vi "PM100D_Initialize.vi"() -> (0 "error out":errorcluster, 1 "Instrument":string, 2 "VISA out":refnum<visa-resource-name>, 4 "SN":string)   [LabVIEW 2010]
doc: "This VI scans for connected devices, that can be selected in a dialog box. Next steps\n- setting timeout\n- performing identification query\n- configuring the operation register to '512'; flag gets to HI when a new measurement value is ready to fetch\n- clear operation register"
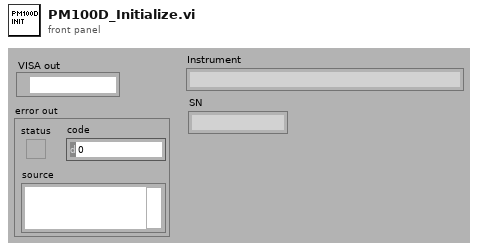
[diagram p1: front panel]
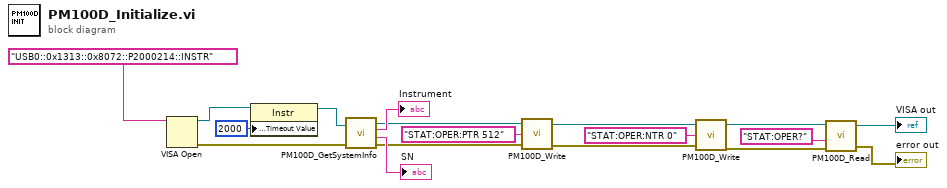
[diagram p0: block diagram]
diagram:
  n1 = VISA Open(VISA resource name="USB0::0x1313::0x8072::P2000214::INSTR" ("element")) -> (VISA resource name=w14:refnum<visa-resource-name>, error out=w18:errorcluster)  [unwired: 1 in, 3 out]
  n2 = property class="Instr"(reference=w14, "General Settings:Timeout Value"=u32 2000) -> (reference out=w13:refnum<visa-resource-name>)  [unwired: 1 in, 1 out]
  n3 = call "PM100D_GetSystemInfo.vi"("VISA in"=w13, "error in"=w18) -> ("VISA out"=w11:refnum<visa-resource-name>, "Instrument"=→"Instrument":string, "SN"=→"SN":string, "error out"=w9:errorcluster)
  n4 = call "PM100D_Write.vi"("error in (no error)"=w9, "Command"="STAT:OPER:PTR 512", "VISA in"=w11) -> ("error out"=w8:errorcluster, "VISA out"=w10:refnum<visa-resource-name>)
  n5 = call "PM100D_Write.vi"("error in (no error)"=w8, "Command"="STAT:OPER:NTR 0", "VISA in"=w10) -> ("error out"=w2:errorcluster, "VISA out"=w6:refnum<visa-resource-name>)
  n6 = call "PM100D_Read.vi"("error in (no error)"=w2, "Command"="STAT:OPER?", "VISA in"=w6) -> ("error out"=→"error out":errorcluster, "VISA out"=→"VISA out":refnum<visa-resource-name>)  [unwired: 2 out]
